vi "Array Split Algorithm.vi"(10 "Modulus":i32, 11 "Array Size":i32) -> (2 "Loop counter":i32)   [LabVIEW 2018, in "PIOD.lvlib" / "PIOD.lvclass"]
uses:
  PIOD.lvclass
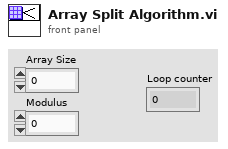
[diagram p1: front panel]
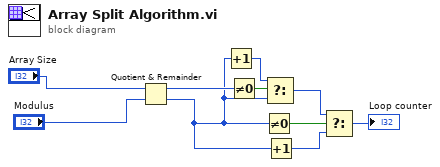
[diagram p0: block diagram]
diagram:
  n1 = Quotient & Remainder(x="Array Size", y="Modulus") -> (x-y*floor(x/y)=w6:i32, floor(x/y)=w4:i32)
  n2 = Increment(x=w4) -> (x+1=w5:i32)
  n3 = Not Equal To 0?(x=w6) -> (x != 0?=w7:bool)
  n4 = Not Equal To 0?(x=w4) -> (x != 0?=w10:bool)
  n5 = Select(t=w5, s=w7, f=w4) -> (s? t:f=w8:i32)
  n6 = Increment(x=w4) -> (x+1=w9:i32)
  n7 = Select(t=w8, s=w10, f=w9) -> (s? t:f=→"Loop counter":i32)
